vi "IVC_OC200_Main.vi"() -> ()   [LabVIEW 2019]
uses:
  IVC_OC200_Global.vi
panel:
  in  "logging_on":bool=TRUE caption="Logging"
  out "status_log":bool caption="Status"
  out "Status":bool
  out "Last Meas. Time":timestamp format="%<%Y-%m-%d %H:%M:%S>T"
  out "chart":waveform(dbl)[](graph)=[{"t0"=timestamp(3785686355.130285 s since 1904-01-01), "dt"=1.0, "Y"=[-0.00251999]}, {"t0"=timestamp(3785686355.130285 s since 1904-01-01), "dt"=1.0, "Y"=[-0.00346989]}]
  out "CH2 (Torr)":dbl
  out "CH1 (Torr)":dbl
  in  "milliseconds to wait":u32=1000
  in  "stop":bool
  in  "VISA resource name":refnum<visa-resource-name>="COM41"
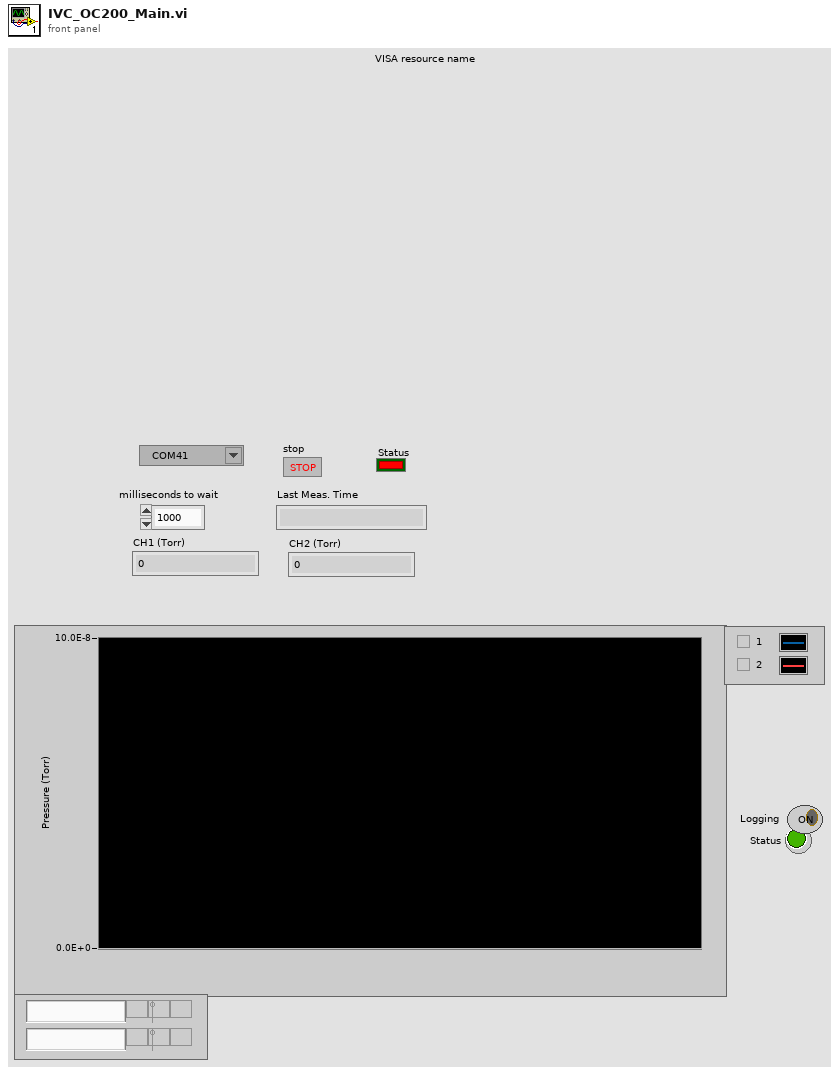
[diagram p1: front panel]
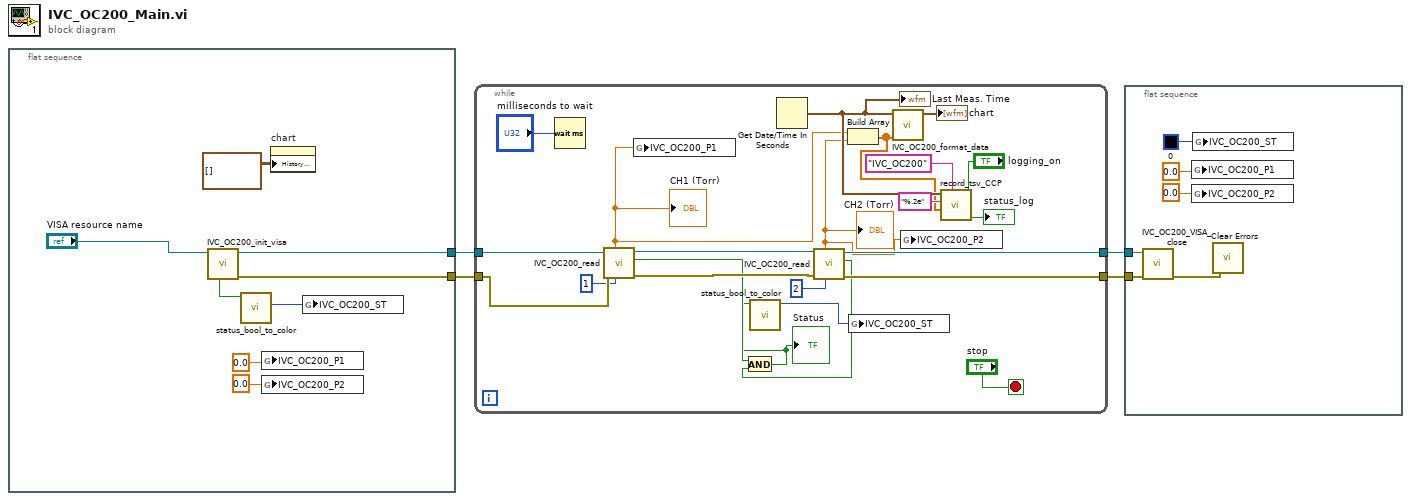
[diagram p0: block diagram]
diagram:
  n1 = flat-sequence {
    tunnel: [w11] -> w4
    tunnel: [w7] -> w3
    frame #0 {
      n2 = call "IVC_OC200_init_visa.vi"("VISA resource name"="VISA resource name") -> ("error out"=w7:errorcluster, "VISA resource name out"=w11:refnum<visa-resource-name>, ".not. x?"=w5:bool)  [unwired: 8 in]
      n3 = call "status_bool_to_color.vi"("status_bool_1"=w5) -> ("status_color"=w6:u32)  [unwired: 10 in]
      n4 = global write "IVC_OC200_Global.vi" "IVC_OC200_P1"(0.0 ("IVC_OC200_P1")) -> ()
      n5 = global write "IVC_OC200_Global.vi" "IVC_OC200_P2"(0.0 ("IVC_OC200_P1")) -> ()
      n6 = property on="chart" class="WFChart (strict)"("History Data"=waveform(dbl)[][] []) -> ()  [unwired: 2 in, 2 out]
      n7 = global write "IVC_OC200_Global.vi" "IVC_OC200_ST"(w6) -> ()
    }
  }
  n8 = while {
    tunnel: w4 -> [w34]
    tunnel: w3 -> [w33]
    tunnel: [w30] -> w2
    tunnel: [w29] -> w1
    stop <- "stop" stop-if-true
    n9 = Wait (ms)(milliseconds to wait="milliseconds to wait") -> ()  [unwired: 1 out]
    n10 = call "IVC_OC200_read.vi"("Channel"=1, "error in (no error)"=w33, "VISA Refnum in"=w34) -> ("error out"=w28:errorcluster, "Status"=w24:bool, "VISA Refnum out"=w31:refnum<visa-resource-name>, "IVC (Torr)"=w16:dbl)  [unwired: 3 in, 2 out]
    "CH1 (Torr)" <- w16
    n11 = global write "IVC_OC200_Global.vi" "IVC_OC200_P1"(w16) -> ()
    n12 = Get Date/Time In Seconds() -> (seconds since 1Jan1904=w21:timestamp)
    "Last Meas. Time" <- w21
    n13 = call "IVC_OC200_read.vi"("Channel"=2, "error in (no error)"=w28, "VISA Refnum in"=w31) -> ("error out"=w30:errorcluster, "Status"=w23:bool, "VISA Refnum out"=w29:refnum<visa-resource-name>, "IVC (Torr)"=w15:dbl)  [unwired: 3 in, 2 out]
    "CH2 (Torr)" <- w15
    n14 = And(x=w24, y=w23) -> (x .and. y?=w13:bool)
    "Status" <- w13
    n15 = call "status_bool_to_color.vi"("status_bool_1"=w13) -> ("status_color"=w14:u32)  [unwired: 10 in]
    n16 = Build Array(w16, w15) -> (w17:dbl[])
    n17 = global write "IVC_OC200_Global.vi" "IVC_OC200_ST"(w14) -> ()
    n18 = call "IVC_OC200_format_data.vi"("element"=w17, "time"=w21) -> ("waveform_array_A"=→"chart":waveform(dbl)[])  [unwired: 9 in]
    n19 = global write "IVC_OC200_Global.vi" "IVC_OC200_P2"(w15) -> ()
    n20 = call "record_tsv_CCP.vi"("logging_on"="logging_on", "folder_name"="IVC_OC200", "value_array"=w17, "format"="%.2e", "time"=w21) -> ("status_log"=→"status_log":bool)  [unwired: 5 in, 1 out]
  }
  n21 = flat-sequence {
    tunnel: w2 -> [w41]
    tunnel: w1 -> [w40]
    frame #0 {
      n22 = call "IVC_OC200_VISA_close.vi"("error in (no error)"=w41, "VISA resource name"=w40) -> ("error out"=w36:errorcluster)  [unwired: 9 in]
      n23 = global write "IVC_OC200_Global.vi" "IVC_OC200_P1"(0.0 ("IVC_OC200_P1")) -> ()
      n24 = global write "IVC_OC200_Global.vi" "IVC_OC200_P2"(0.0 ("IVC_OC200_P1")) -> ()
      n25 = global write "IVC_OC200_Global.vi" "IVC_OC200_ST"(u32 0 ("MKS670_1000_ST")) -> ()
      n26 = call <vilib>:"Clear Errors.vi"("error in (no error)"=w36) -> ()  [unwired: 5 in, 2 out]
    }
  }
